vi "FTW-SEQ-Construct.vi"(1 "Initial Sequence":string) -> (0 "FTW Job Sequencer":refnum<class "FTW-JobSequencer.lvclass">)   [LabVIEW 2012, in "FTW-Actor.lvlib" / "FTW-JobSequencer.lvclass"]
uses:
  FTW-JobSequencer.lvclass
  FTW-JobSequencer.lvclass/FTW-JobSequencer.ctl
panel:
  # "Inputs"
  # "Outputs"
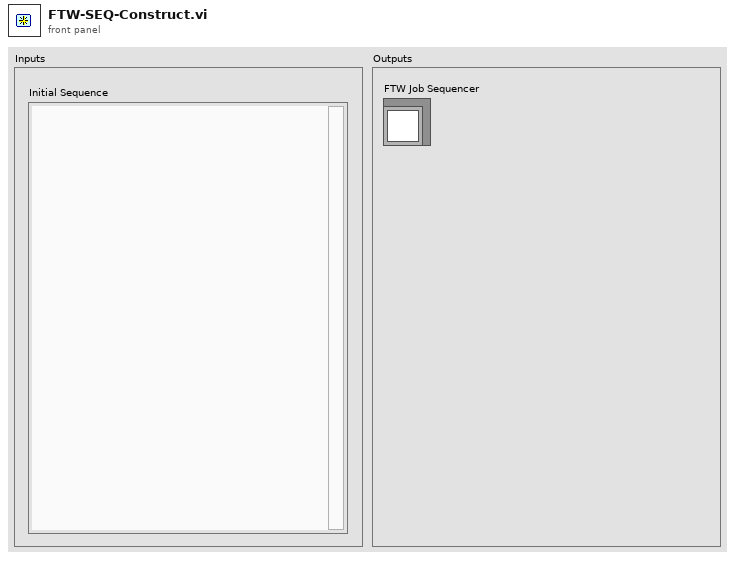
[diagram p1: front panel]
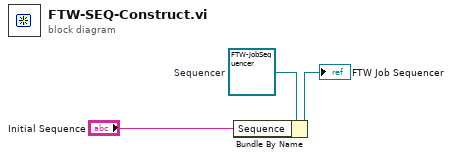
[diagram p0: block diagram]
diagram:
  w3 = refnum<class "FTW-JobSequencer.lvclass"> refnum  # Sequencer
  n1 = Bundle By Name(cluster=w3, "Sequence"="Initial Sequence") -> (→"FTW Job Sequencer":refnum<class "FTW-JobSequencer.lvclass">)
